vi "sub_SDR_mimo_equalizer.vi"(7 "Symbols per Pilot":i32=16, 8 "Input Symbols Port 2":cdb[](array[numeric]), 10 "Input Symbols Port 1":cdb[](array[numeric])) -> (0 "Output symbols Port 2":cdb[](array[numeric]), 3 "Output symbols Port 1":cdb[](array[numeric]), 4 "SNR Before Equalizer":dbl[](array[numeric]))   [LabVIEW 2012]
uses:
  <vilib>/Analysis/2dsp.llb/Decimate (single shot, CDB).vi
  <vilib>/Analysis/2dsp.llb/Upsample (CDB).vi
  <vilib>/Analysis/2dsp.llb/1D Convolution (CDB).vi
  <vilib>/Analysis/NI_AALPro.lvlib
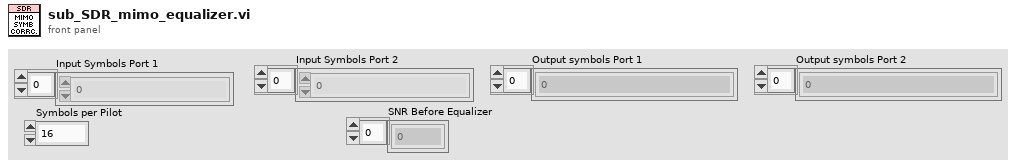
[diagram p1: front panel]
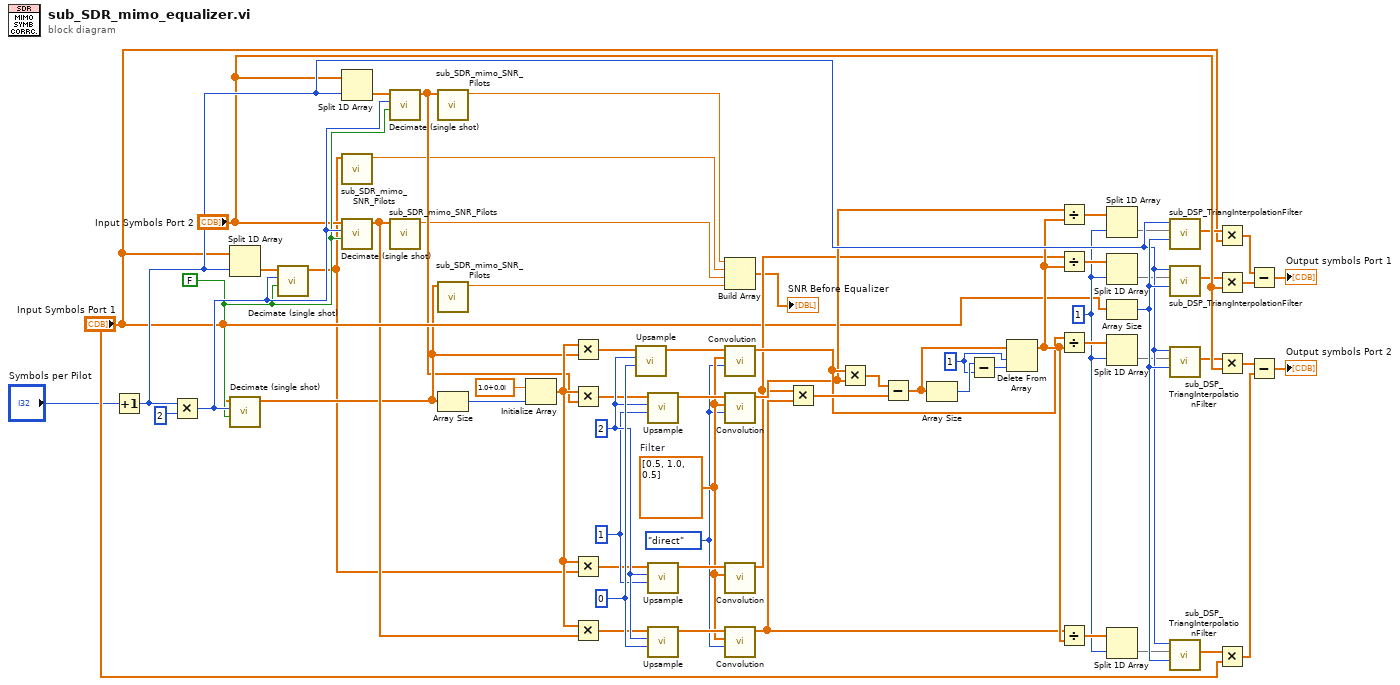
[diagram p0: block diagram]
diagram:
  w27 = 1 ("length")
  w39 = 1 ("index")
  w55 = 1 ("leading zeros")
  w52 = enum32{"direct", "frequency domain"}."direct" ("algorithm")
  w53 = dbl[] [0.5, 1.0, 0.5]  # Filter
  w62 = 0 ("leading zeros")
  w56 = 2 ("upsampling factor")
  w57 = FALSE ("averaging")
  n1 = Increment(x="Symbols per Pilot") -> (x+1=w46:i32)
  n2 = Multiply(x=w46, y=2) -> (x*y=w58:i32)
  n3 = Split 1D Array(array="Input Symbols Port 1", index=w46) -> (second subarray=w60:cdb[])  [unwired: 1 out]
  n4 = call-poly <vilib>:"Decimate (single shot).vi"("averaging"=w57, "decimating factor"=w58, "X"="Input Symbols Port 1") -> ("Decimated Array"=w8:cdb[])  [unwired: 7 in, 1 out]
  n5 = call-poly <vilib>:"Decimate (single shot).vi"("averaging"=w57, "decimating factor"=w58, "X"=w60) -> ("Decimated Array"=w7:cdb[])  [unwired: 7 in, 1 out]
  n6 = Split 1D Array(array="Input Symbols Port 2", index=w46) -> (second subarray=w59:cdb[])  [unwired: 1 out]
  n7 = call "sub_SDR_mimo_SNR_Pilots.vi"("Decimated Array"=w7) -> ("SNR (dB)"=w4:dbl)  [unwired: 10 in]
  n8 = call-poly <vilib>:"Decimate (single shot).vi"("averaging"=w57, "decimating factor"=w58, "X"="Input Symbols Port 2") -> ("Decimated Array"=w9:cdb[])  [unwired: 7 in, 1 out]
  n9 = call-poly <vilib>:"Decimate (single shot).vi"("averaging"=w57, "decimating factor"=w58, "X"=w59) -> ("Decimated Array"=w6:cdb[])  [unwired: 7 in, 1 out]
  n10 = call "sub_SDR_mimo_SNR_Pilots.vi"("Decimated Array"=w9) -> ("SNR (dB)"=w3:dbl)  [unwired: 10 in]
  n11 = call "sub_SDR_mimo_SNR_Pilots.vi"("Decimated Array"=w6) -> ("SNR (dB)"=w5:dbl)  [unwired: 10 in]
  n12 = call "sub_SDR_mimo_SNR_Pilots.vi"("Decimated Array"=w8) -> ("SNR (dB)"=w2:dbl)  [unwired: 10 in]
  n13 = Array Size(array=w8) -> (size(s)=w17:i32)
  n14 = Initialize Array(cdb 1.0+0.0i ("element"), w17) -> (w11:cdb[])
  n15 = Multiply(x=w11, y=w8) -> (x*y=w15:cdb[])
  n16 = Multiply(x=w11, y=w6) -> (x*y=w12:cdb[])
  n17 = Multiply(x=w11, y=w7) -> (x*y=w14:cdb[])
  n18 = Multiply(x=w11, y=w9) -> (x*y=w13:cdb[])
  n19 = call-poly <vilib>:"Upsample.vi"("leading zeros"=w62, "upsampling factor"=w56, "X"=w15) -> ("Upsampled Array"=w64:cdb[])  [unwired: 7 in, 1 out]
  n20 = call-poly <vilib>:"Upsample.vi"("leading zeros"=w55, "upsampling factor"=w56, "X"=w12) -> ("Upsampled Array"=w54:cdb[])  [unwired: 7 in, 1 out]
  n21 = call-poly <vilib>:"Upsample.vi"("leading zeros"=w55, "upsampling factor"=w56, "X"=w14) -> ("Upsampled Array"=w61:cdb[])  [unwired: 7 in, 1 out]
  n22 = call-poly <vilib>:"Upsample.vi"("leading zeros"=w62, "upsampling factor"=w56, "X"=w13) -> ("Upsampled Array"=w63:cdb[])  [unwired: 7 in, 1 out]
  n23 = Build Array(w5, w4, w3, w2) -> (→"SNR Before Equalizer":dbl[])
  n24 = call-poly <vilib>:"Convolution.vi"("algorithm"=w52, "Y"=w53, "X"=w64) -> ("X * Y"=w22:cdb[])  [unwired: 7 in, 1 out]
  n25 = call-poly <vilib>:"Convolution.vi"("algorithm"=w52, "Y"=w53, "X"=w54) -> ("X * Y"=w21:cdb[])  [unwired: 7 in, 1 out]
  n26 = call-poly <vilib>:"Convolution.vi"("Y"=w53, "X"=w61) -> ("X * Y"=w19:cdb[])  [unwired: 8 in, 1 out]
  n27 = call-poly <vilib>:"Convolution.vi"("algorithm"=w52, "Y"=w53, "X"=w63) -> ("X * Y"=w20:cdb[])  [unwired: 7 in, 1 out]
  n28 = Multiply(x=w19, y=w20) -> (x*y=w50:cdb[])
  n29 = Multiply(x=w22, y=w21) -> (x*y=w51:cdb[])
  n30 = Subtract(x=w51, y=w50) -> (x-y=w25:cdb[])
  n31 = Array Size(array=w25) -> (size(s)=w28:i32)
  n32 = Subtract(x=w28, y=w27) -> (x-y=w26:i32)
  n33 = Delete From Array(array=w25, length=w27, index=w26) -> (array with subset deleted=w29:cdb[])  [unwired: 1 out]
  n34 = Divide(x=w21, y=w29) -> (x/y=w24:cdb[])
  n35 = Divide(x=w19, y=w29) -> (x/y=w41:cdb[])
  n36 = Divide(x=w22, y=w29) -> (x/y=w43:cdb[])
  n37 = Divide(x=w20, y=w29) -> (x/y=w40:cdb[])
  n38 = Split 1D Array(array=w24, index=w39) -> (second subarray=w30:cdb[])  [unwired: 1 out]
  n39 = Split 1D Array(array=w41, index=w39) -> (second subarray=w42:cdb[])  [unwired: 1 out]
  n40 = Array Size(array="Input Symbols Port 1") -> (size(s)=w47:i32)
  n41 = Split 1D Array(array=w43, index=w39) -> (second subarray=w36:cdb[])  [unwired: 1 out]
  n42 = Split 1D Array(array=w40, index=w39) -> (second subarray=w38:cdb[])  [unwired: 1 out]
  n43 = call "sub_DSP_TriangInterpolationFilter.vi"("Desired Len"=w47, "X"=w30, "Interpolation factor"=w46) -> ("Interpolated X"=w34:cdb[])  [unwired: 8 in]
  n44 = call "sub_DSP_TriangInterpolationFilter.vi"("Desired Len"=w47, "X"=w42, "Interpolation factor"=w46) -> ("Interpolated X"=w33:cdb[])  [unwired: 8 in]
  n45 = call "sub_DSP_TriangInterpolationFilter.vi"("Desired Len"=w47, "X"=w36, "Interpolation factor"=w46) -> ("Interpolated X"=w31:cdb[])  [unwired: 8 in]
  n46 = call "sub_DSP_TriangInterpolationFilter.vi"("Desired Len"=w47, "X"=w38, "Interpolation factor"=w46) -> ("Interpolated X"=w32:cdb[])  [unwired: 8 in]
  n47 = Multiply(x=w34, y="Input Symbols Port 1") -> (x*y=w45:cdb[])
  n48 = Multiply(x=w33, y="Input Symbols Port 2") -> (x*y=w49:cdb[])
  n49 = Multiply(x=w31, y="Input Symbols Port 2") -> (x*y=w37:cdb[])
  n50 = Multiply(x=w32, y="Input Symbols Port 1") -> (x*y=w48:cdb[])
  n51 = Subtract(x=w45, y=w49) -> (x-y=→"Output symbols Port 1":cdb[])
  n52 = Subtract(x=w37, y=w48) -> (x-y=→"Output symbols Port 2":cdb[])
